vi "Update UI.vi"(7 "Message (Value Change)":string="Value Change", 8 "error in (no error)":errorcluster, 9 "Data":variant, 10 "Target":string, 11 "ID":string) -> (0 "error out":errorcluster)   [LabVIEW 2019, in "Messaging.lvlib"]
doc: "Simple wrapper for sending messages to the UI. If Message is not specified, the default message is a Value Change."
uses:
  Messaging.lvlib
  Message Cluster.ctl
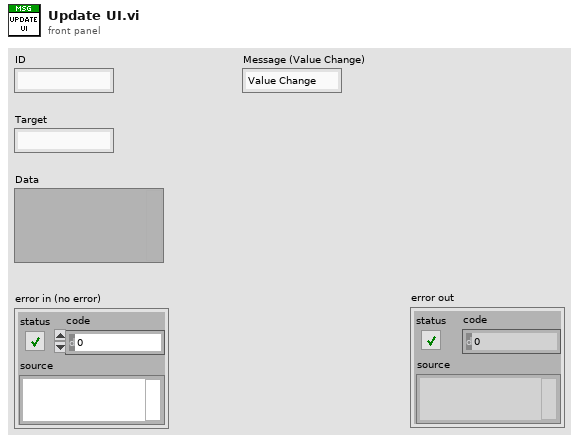
[diagram p1: front panel]
types:
  T1 = typedef "Messaging.lvlib/Message Cluster.ctl" = cluster{"Event":string, "Source":string, "Target":string, "Data":variant}
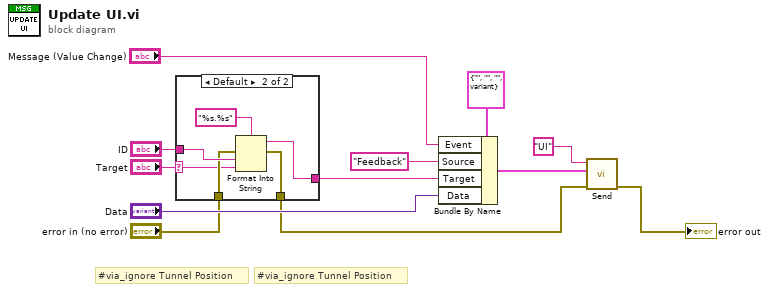
[diagram p0: block diagram]
diagram:
  # "#via_ignore Tunnel Position"
  # "#via_ignore Tunnel Position"
  n1 = case shown="Default" "Target" {
    selector: "Target" -> [_ w15]
    tunnel: "ID" -> [w14 w20]
    tunnel: [w14 w18] -> w9
    tunnel: "error in (no error)" -> [w13 w17]
    tunnel: [w13 w16] -> w3
    frame "" {
    }
    frame Default {
      n2 = Format Into String(format string="%s.%s", error in=w17, w20, w15) -> (resulting string=w18:string, error out=w16:errorcluster)  [unwired: 1 in]
    }
  }
  n3 = Bundle By Name(cluster=T1 {"Event"="", "Source"="", "Target"="", "Data"=variant} ("Message"), "Event"="Message (Value Change)", "Source"="Feedback", "Target"=w9, "Data"="Data") -> (w7:T1)
  n4 = call "Send.vi"("error in (no error)"=w3, "Message"=w7, "Queue Name"="UI") -> ("error out"=→"error out":errorcluster)  [unwired: 8 in]
